vi "Labview and RPI interface.vi"() -> ()   [LabVIEW 2025]
panel:
  in  "Stop":bool
  out "Chlol-a":dbl
  out "SST":dbl
  out "Longitude":dbl
  out "Latitude":dbl
  # "Sensors Data"
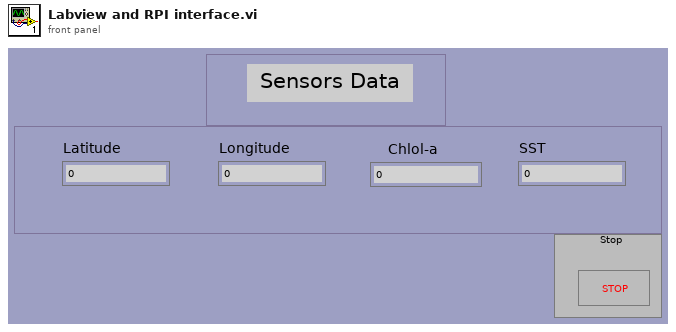
[diagram p1: front panel]
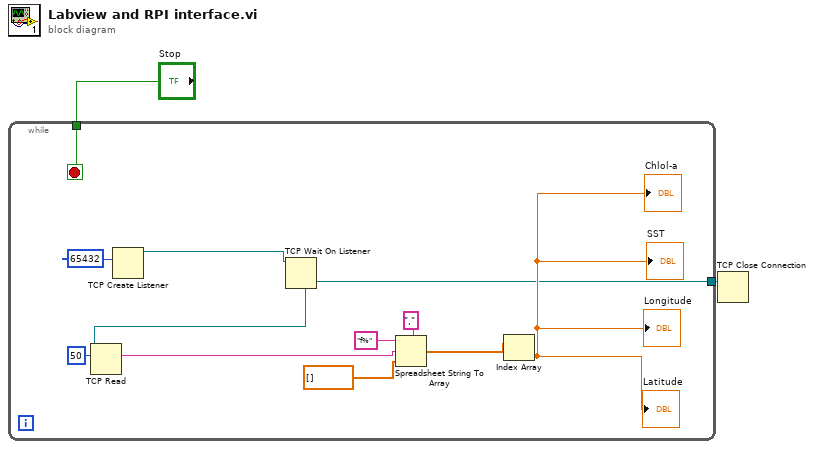
[diagram p0: block diagram]
diagram:
  n1 = while {
    tunnel: [w6] -> w2
    tunnel: "Stop" -> [w5]
    stop <- w5 stop-if-true
    n2 = TCP Create Listener(10:u16 65432 ("port")) -> (3:w12:refnum<k5>)  [unwired: 4 in, 2 out]
    n3 = TCP Wait On Listener(11:w12) -> (4:w6:refnum<k5>)  [unwired: 3 in, 4 out]
    n4 = TCP Read(connection ID=w6, bytes to read=50) -> (data out=w4:string)  [unwired: 3 in, 2 out]
    n5 = Spreadsheet String To Array(delimiter (Tab)=",", format string="f%", spreadsheet string=w4, array type (2D Dbl)=dbl[] []) -> (array=w9:dbl[])
    n6 = Index Array(array=w9) -> (element=→"Chlol-a" →"SST" →"Longitude" →"Latitude":dbl)  [unwired: 1 in]
  }
  n7 = TCP Close Connection(connection ID=w2) -> ()  [unwired: 2 in, 2 out]
